vi "Convert Polar To  to XY Velocties.vi"(11 "Traverse":T2 {"Angle" scale format="%.3f"; "Velocity" scale=-1.0..1.0 scale format="%.1f"}) -> (3 "XY Velocities Out":T1)   [LabVIEW 2023, in "Thor-SwerveDrive_ACT.lvlib"]
uses:
  Thor-SwerveDrive_ACT.lvlib
  Shared Code/TypeDefs/Cluster_Module Velocity-Direction-Rotations.ctl
  Shared Code/TypeDefs/Level_Velocity plus-minus 1.ctl
  Shared Code/TypeDefs/Dial_Compase heading unit circle CCW positive.ctl
  Shared Code/TypeDefs/Cluster_X-Y.ctl
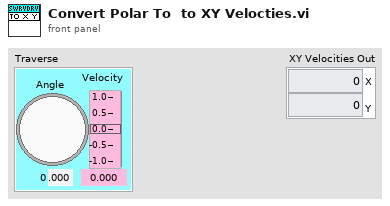
[diagram p1: front panel]
types:
  T1 = typedef "Cluster_X-Y.ctl" = cluster{"X":dbl, "Y":dbl}
  T2 = typedef "Cluster_Module Velocity-Direction-Rotations.ctl" = cluster{"Velocity":T3, "Angle":T4, "Rotations Count":dbl}
  T3 = typedef "Level_Velocity plus-minus 1.ctl" = dbl
  T4 = typedef "Dial_Compase heading unit circle CCW positive.ctl" = dbl
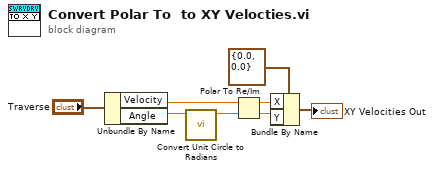
[diagram p0: block diagram]
diagram:
  n1 = Unbundle By Name("Traverse") -> ("Velocity"=w7:T3, "Angle"=w5:T4)
  n2 = call "Convert Unit Circle to Radians.vi"("Unit Circle"=w5) -> ("Radians"=w6:dbl)  [unwired: 10 in]
  n3 = Polar To Re/Im(2:w6, 3:w7) -> (0:w3:T3, 1:w2:T3)
  n4 = Bundle By Name(cluster=T1 {"X"=0.0, "Y"=0.0} ("XY"), "X"=w2, "Y"=w3) -> (→"XY Velocities Out":T1)
